vi "Handle Messages.vi"(8 "error in (no error)":errorcluster, 9 "Message Data":variant, 10 "Message":string, 11 "Cashier In":refnum<class "Cashier.lvclass">) -> (0 "error out":errorcluster, 3 "Cashier Out":refnum<class "Cashier.lvclass">)   [LabVIEW 2020, in "Cashier.lvclass"]
uses:
  Cashier.lvclass
  C:/Users/anton/Documents/GitHub/Triarc-Examples/Coffee Shop/Person/Person.lvclass
  Support/Order/Order.lvclass
  Worker/Worker.lvclass
  Customers/Customer/Customer.lvclass
  Person/Person.lvclass
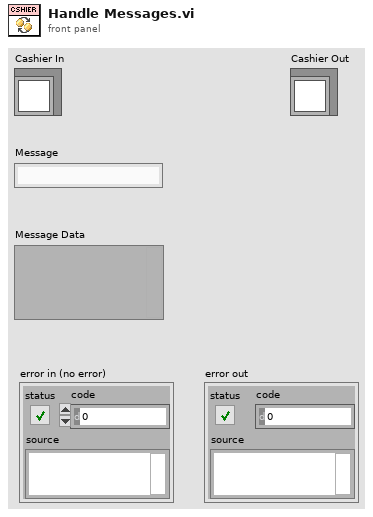
[diagram p1: front panel]
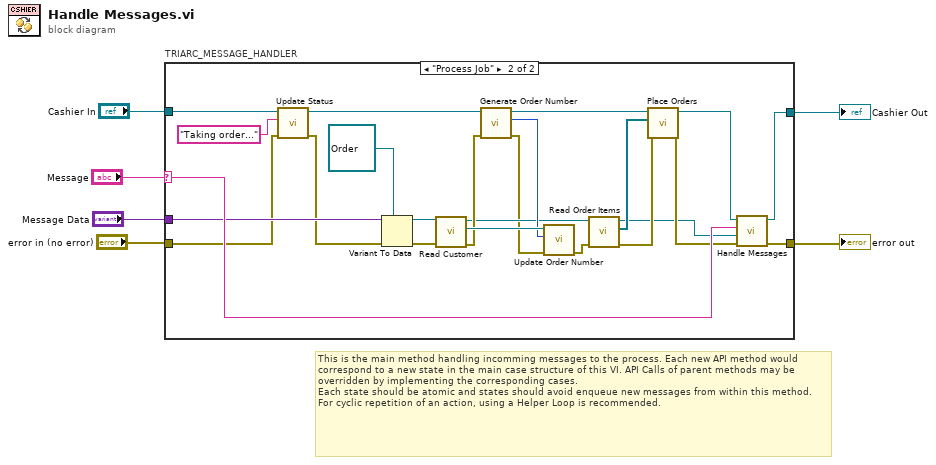
[diagram p0: block diagram]
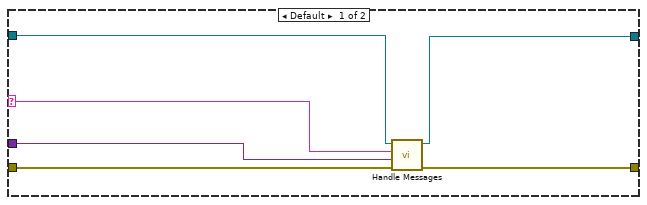
[diagram p2: hidden frame]
diagram:
  # "This is the main method handling incomming messages to the process. Each new API method would correspond to a new state in the main case structure of this VI. API Calls of parent methods may be overridden by implementing the corresponding cases.\nEach state should be atomic and states should avoid enqueue new messages from within this method. For cyclic repetition of an action, using a Helper Loop is recommended."
  n1 = case "TRIARC_MESSAGE_HANDLER" shown="\"Process Job\"" "Message" {
    selector: "Message" -> [w10 w35]
    tunnel: "error in (no error)" -> [w9 w28]
    tunnel: "Cashier In" -> [w12 w36]
    tunnel: "Message Data" -> [w11 w32]
    tunnel: [w8 w34] -> w2
    tunnel: [w7 w33] -> w1
    frame Default {
      n2 = call-parent "Handle Messages.vi"("error in (no error)"=w9, "Message Data"=w11, "Message"=w10, "Worker In"=w12) -> ("error out"=w8:errorcluster, "Worker Out"=w7:refnum<class "Cashier.lvclass">)  [unwired: 6 in]
    }
    frame "Process Job" {
      n3 = call "Update Status.vi"("error in (no error)"=w28, "Status"="Taking order..." ("Message"), "Person In"=w36) -> ("error out"=w29:errorcluster, "Person Out"=w30:refnum<class "Cashier.lvclass">)  [unwired: 7 in]
      n4 = Variant To Data(error in=w29, type=refnum<class "Order.lvclass"> refnum ("Order.lvclass"), Variant=w32) -> (data=w27:refnum<class "Order.lvclass">, error out=w24:errorcluster)
      n5 = call-dynamic "Read Customer.vi"("error in (no error)"=w24, "Order in"=w27) -> ("error out"=w23:errorcluster, "Customer"=w26:refnum<class "Customer.lvclass">, "Order out"=w22:refnum<class "Order.lvclass">)  [unwired: 7 in]
      n6 = call "Generate Order Number.vi"("error in (no error)"=w23, "Cashier in"=w30) -> ("error out"=w21:errorcluster, "Order Number"=w25:u32, "Cashier out"=w19:refnum<class "Cashier.lvclass">)  [unwired: 7 in]
      n7 = call "Update Order Number.vi"("error in (no error)"=w21, "Order Number"=w25, "Customer In"=w26) -> ("error out"=w20:errorcluster)  [unwired: 7 in, 1 out]
      n8 = call-dynamic "Read Order Items.vi"("error in (no error)"=w20, "Order in"=w22) -> ("error out"=w15:errorcluster, "Items"=w17:refnum<class "Order Item.lvclass">[], "Order out"=w14:refnum<class "Order.lvclass">)  [unwired: 7 in]
      n9 = call "Place Orders.vi"("error in (no error)"=w15, "Items"=w17, "Cashier in"=w19) -> ("error out"=w16:errorcluster, "Cashier out"=w18:refnum<class "Cashier.lvclass">)  [unwired: 7 in]
      n10 = call-parent "Handle Messages.vi"("error in (no error)"=w16, "Message Data"=w14, "Message"=w35, "Worker In"=w18) -> ("error out"=w34:errorcluster, "Worker Out"=w33:refnum<class "Cashier.lvclass">)  [unwired: 6 in]
    }
  }
  "error out" <- w2
  "Cashier Out" <- w1
